vi "Ballard - Arinc-429 RT Driver VI old old.vi"(7 "Operation":T1, 11 "Device Reference in":T2 format="%.0x") -> (0 "Error Code":i32)   [LabVIEW 2016, in "Ballard Arinc-429 Engine.lvlib"]
uses:
  Ballard Arinc-429 Engine.lvlib
  RT Controls/Async Loop Control Enum.ctl
  RT Controls/ReadWrite Selector.ctl
  Shared/Controls and Global/Label.ctl
  Shared/Ballard Arinc-429 Shared.lvlib
  Shared/Controls and Global/transferPeriod.ctl
  <vilib>/NI Veristand/Custom Device API/Data Reference.ctl
  <vilib>/NI Veristand/Custom Device API/Custom Device API.lvlib
  <vilib>/NI Veristand/Custom Device API/Block Data Reference.ctl
  Shared/Controls and Global/Start Bit.ctl
  Shared/Controls and Global/Number of Bits.ctl
  RT Controls/Driver Data.ctl
  RT Controls/RT Label Settings.ctl
  RT Controls/RT HW Channel.ctl
  RT Controls/Error Qs.ctl
  RT Controls/Status Channels Config.ctl
  RT Controls/FIFO.ctl
  RT Controls/Label Transfer Config.ctl
  RT Controls/RT Data.ctl
  RT Controls/RT Param Setting.ctl
  RT Controls/RT Word Settings.ctl
  Shared/Controls and Global/TransferType.ctl
  <vilib>/NI Veristand/Custom Device API/Custom Device Item Ref.ctl
  <vilib>/NI Veristand/Custom Device API/Hardware Interface Driver VI Operation.ctl
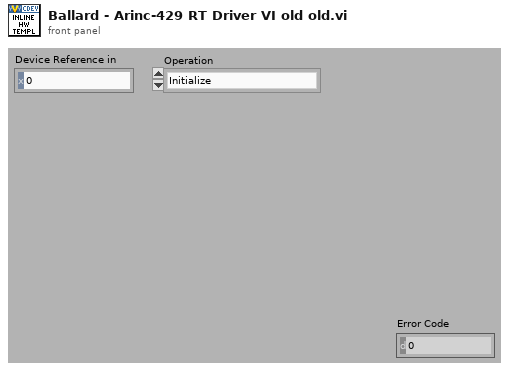
[diagram p1: front panel]
types:
  T1 = typedef "Custom Device API.lvlib/Hardware Interface Driver VI Operation.ctl" = enum16{"Initialize", "Start", "Read Data from HW", "Write Data to HW", "Close"}
  T2 = typedef "Custom Device API.lvlib/Custom Device Item Ref.ctl" = u64
  T3 = typedef "Ballard Arinc-429 Engine.lvlib/RT Data.ctl" = cluster{"HWInput Channels":T4[], "HWOutput Channels":T4[], "board handle":u32, "Start":refnum<notifier>, "HWIn BaseRate":i64, "HWOut BaseRate":i64, "Error Qs":T16, "Error Pub Q":refnum<queue>, "Status Config":T17, "FIFOs":T18, "VI Refs":refnum<vi>[], "Label Transfer Config":T19, "ScheduledSDI":bool}
  T4 = typedef "Ballard Arinc-429 Engine.lvlib/RT HW Channel.ctl" = cluster{"Labels Settings":T5[], "channel handle":u32, "channel #":u16, "Label Map":i32[], "Label Buffer":u32[], "rdBufHandle":u32}
  T5 = typedef "Ballard Arinc-429 Engine.lvlib/RT Label Settings.ctl" = cluster{"Name":string, "xmlName":string, "Label":T6, "transferPeriod":T7, "Driver Data":T8, "SDI_Enabled":bool, "SDI":u8, "Words":T9[], "bufferSize":u32, "RxWordIdx":i32, "TxWordIdx":i32, "TransferType":T15, "has timestamp?":bool}
  T6 = typedef "Ballard Arinc-429 Shared.lvlib/Label.ctl" = u8
  T7 = typedef "Ballard Arinc-429 Shared.lvlib/transferPeriod.ctl" = u32
  T8 = typedef "Ballard Arinc-429 Engine.lvlib/Driver Data.ctl" = cluster{"Lbl Tx Hdl":u32, "Decimation":i32, "IterationOffset":i32, "transfer handle":u32, "RX Word":u32, "TXChange":bool, "RX timestamp":dbl}
  T9 = typedef "Ballard Arinc-429 Engine.lvlib/RT Word Settings.ctl" = cluster{"Block Data Refs":T10[], "Values Array":dbl[], "Length":i32, "FIFO Index":i32, "Param Setting":T12}
  T10 = typedef "Custom Device API.lvlib/Block Data Reference.ctl" = cluster{"Data Reference":T11, "Offset":u64, "Length":u64}
  T11 = typedef "Custom Device API.lvlib/Data Reference.ctl" = i32
  T12 = typedef "Ballard Arinc-429 Engine.lvlib/RT Param Setting.ctl" = cluster{"Start Bit":T13[], "Num Bits":T14[], "Signed?":bool[], "ScaleFac":dbl[], "ScaleOffset":dbl[]}
  T13 = typedef "Ballard Arinc-429 Shared.lvlib/Start Bit.ctl" = i32
  T14 = typedef "Ballard Arinc-429 Shared.lvlib/Number of Bits.ctl" = i32
  T15 = typedef "Ballard Arinc-429 Shared.lvlib/TransferType.ctl" = enum16{"ScheduledLabel", "Acyclic", "Block", "Strobe"}
  T16 = typedef "Ballard Arinc-429 Engine.lvlib/Error Qs.ctl" = cluster{"HWIn":refnum<queue>, "HWOut":refnum<queue>, "TransCfg":refnum<queue>}
  T17 = typedef "Ballard Arinc-429 Engine.lvlib/Status Channels Config.ctl" = cluster{"Error Data Ref":T11, "HWIn Dur Ref":T11, "HWIn Dur Idx":i32, "HWOut Dur Ref":T11, "HWOut Dur Idx":i32}
  T18 = typedef "Ballard Arinc-429 Engine.lvlib/FIFO.ctl" = cluster{"From HWIn":refnum<k33>, "To HWOut":refnum<k33>, "From HWIn Buf":dbl[], "To HWOut Buf":dbl[], "To TansCfg":refnum<k33>, "To TransCfg Buf":dbl[], "From HWOut":refnum<k33>, "From HWOut Buf":dbl[], "Old To HWOut Buf":dbl[]}
  T19 = typedef "Ballard Arinc-429 Engine.lvlib/Label Transfer Config.ctl" = cluster{"Block Data Refs":T10[], "Values Array":dbl[]}
  T20 = typedef "Ballard Arinc-429 Engine.lvlib/Async Loop Control Enum.ctl" = enum16{"Launch", "Start", "Stop"}
  T21 = typedef "Ballard Arinc-429 Engine.lvlib/ReadWrite Selector.ctl" = enum16{"Inline Read", "Inline Write", "Async HWIn", "Async HWOut"}
  T22 = typedef "Ballard Arinc-429 Engine.lvlib/FIFO Idx Qs.ctl" = cluster{"From HWInput":refnum<queue>, "To HWOutput":refnum<queue>, "From HWOutput":refnum<queue>}
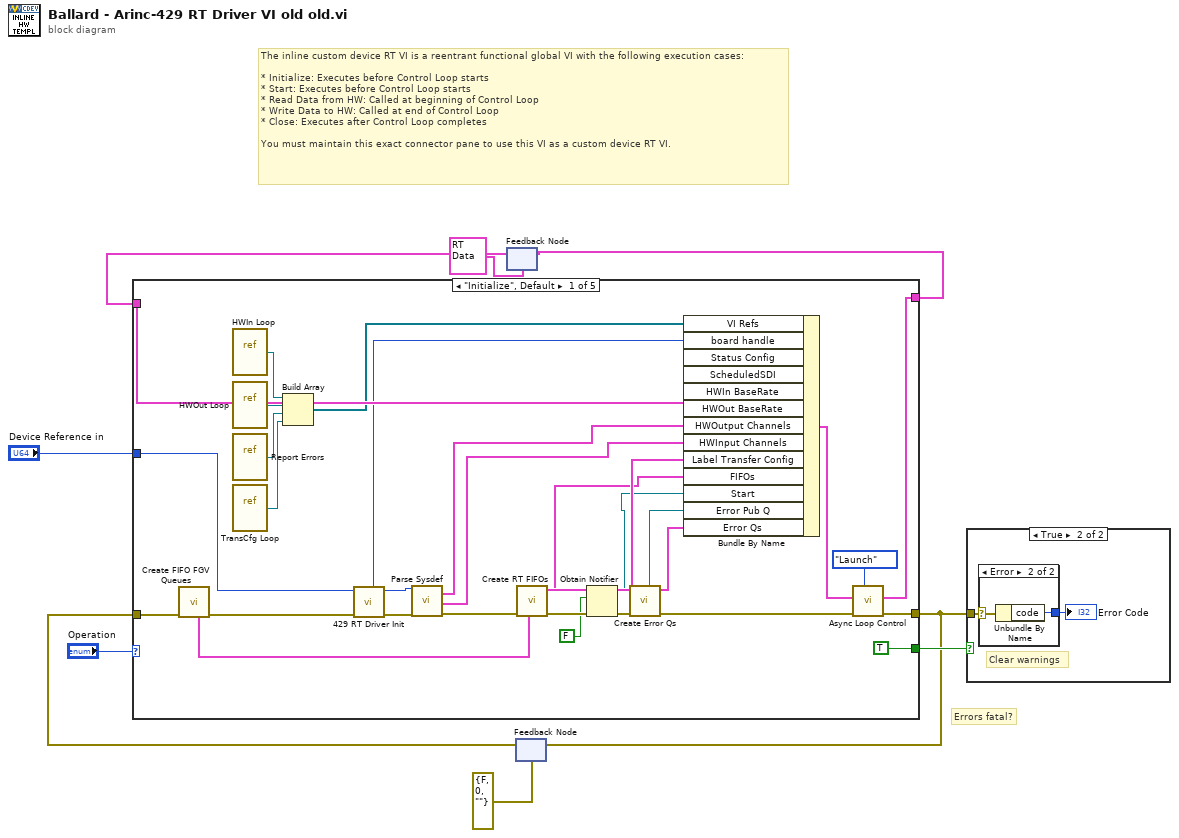
[diagram p0: block diagram]
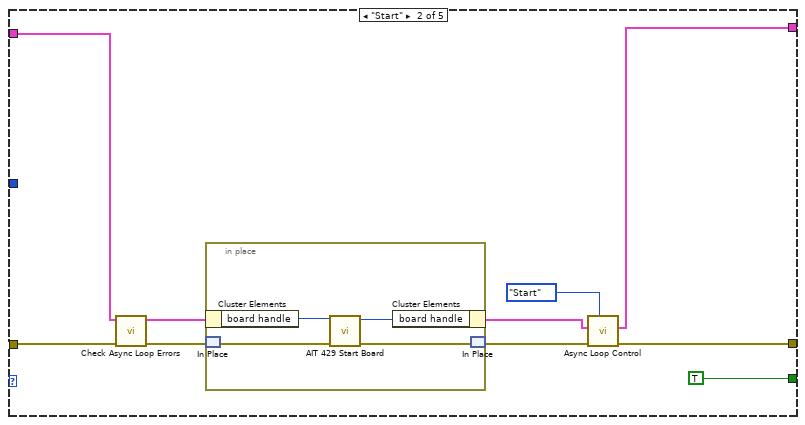
[diagram p4: hidden frame]
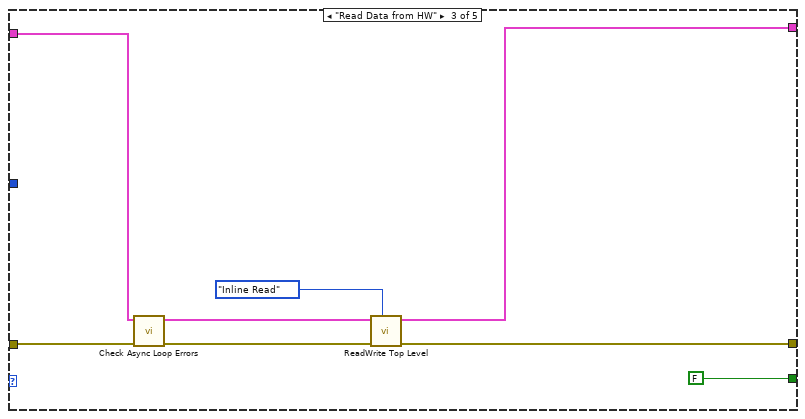
[diagram p5: hidden frame]
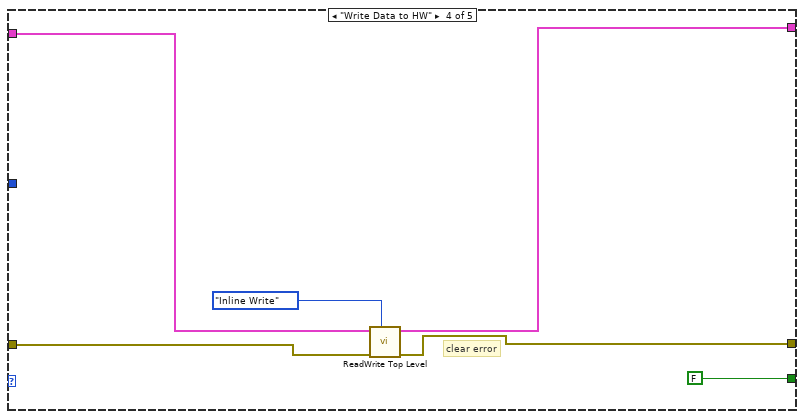
[diagram p6: hidden frame]
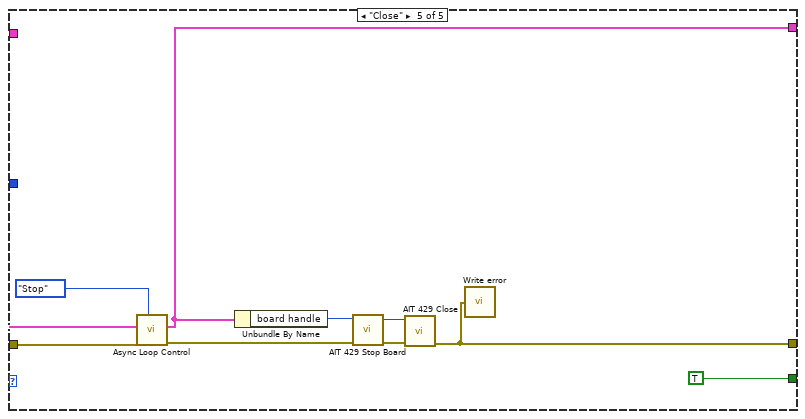
[diagram p7: hidden frame]
diagram:
  # "Errors fatal?"
  # "The inline custom device RT VI is a reentrant functional global VI with the following execution cases:\n\n* Initialize: Executes before Control Loop starts\n* Start: Executes before Control Loop starts\n* Read Data from HW: Called at beginning of Control Loop\n* Write Data to HW: Called at end of Control Loop\n* Close: Executes after Control Loop completes\n\nYou must maintain this exact connector pane to use this VI as a custom device RT VI."
  n1 = feedback #1(T3 {"HWInput Channels"=[], "HWOutput Channels"=[], "board handle"=0, "Start"=refnum, "HWIn BaseRate"=0, "HWOut BaseRate"=0, "Error Qs"={"HWIn"=refnum, "HWOut"=refnum, "TransCfg"=refnum}, "Error Pub Q"=refnum, "Status Config"={"Error Data Ref"=0, "HWIn Dur Ref"=0, "HWIn Dur Idx"=0, "HWOut Dur Ref"=0, "HWOut Dur Idx"=0}, "FIFOs"={"From HWIn"=refnum, "To HWOut"=refnum, "From HWIn Buf"=[], "To HWOut Buf"=[], "To TansCfg"=refnum, "To TransCfg Buf"=[], "From HWOut"=refnum, "From HWOut Buf"=[], "Old To HWOut Buf"=[]}, "VI Refs"=[], "Label Transfer Config"={"Block Data Refs"=[], "Values Array"=[]}, "ScheduledSDI"=FALSE} ("RT Data")) -> (w4:T3)
  n2 = feedback #2(errorcluster {"status"=FALSE, "code"=0, "source"=""} ("error out")) -> (w2:errorcluster)
  n3 = case shown="\"Initialize\", Default" "Operation" {
    tunnel: w4 -> [w29 w51 w62 w71 w76]
    tunnel: "Device Reference in" -> [w31 _ _ _ _]
    tunnel: [w37 w44 w64 w70 w75] -> w3
    tunnel: [w41 w52 w65 w66 w79] -> w1
    tunnel: w2 -> [w11 w50 w59 w69 w78]
    tunnel: [TRUE TRUE FALSE FALSE TRUE] -> w7
    frame "Initialize", Default {
      n4 = call "Create FIFO FGV Queues.vi"("error in (no error)"=w11) -> ("error out"=w13:errorcluster, "FIFO Idx Qs"=w36:T22)  [unwired: 9 in]
      n5 = vi-ref "HWIn Loop.vi"() -> (w33:refnum<vi>)
      n6 = vi-ref "HWOut Loop.vi"() -> (w34:refnum<vi>)
      n7 = vi-ref "Report Errors.vi"() -> (w35:refnum<vi>)
      n8 = vi-ref "TransCfg Loop.vi"() -> (w32:refnum<vi>)
      n9 = Build Array(w33, w34, w35, w32) -> (w27:refnum<vi>[])
      n10 = call "429 RT Driver Init.vi"("error in"=w13, "Device Reference in"=w31) -> ("error out"=w12:errorcluster, "Device Reference out"=w30:T2, "board handle"=w26:u32)  [unwired: 5 in, 2 out]
      n11 = call "Parse Sysdef.vi"("Device Reference in"=w30, "error in (no error)"=w12) -> ("HWOutput Section Data"=w20:T4[], "HWInput Section Data"=w19:T4[], "error out"=w25:errorcluster)  [unwired: 10 in, 5 out]
      n12 = call "Create RT FIFOs.vi"("FIFO Idx Qs"=w36, "error in (no error)"=w25) -> ("error out"=w43:errorcluster, "output cluster"=w17:T18, "Label Transfer Config"=w18:T19)  [unwired: 7 in]
      n13 = Obtain Notifier(notification data type=FALSE, error in (no error)=w43) -> (notifier out=w16:refnum<notifier>, error out=w39:errorcluster)  [unwired: 2 in, 1 out]
      n14 = call "Create Error Qs.vi"("error in (no error)"=w39) -> ("error out"=w10:errorcluster, "Error Qs"=w14:T16, "Error Publishing Q"=w15:refnum<queue>)  [unwired: 8 in]
      n15 = Bundle By Name(cluster=w29, "VI Refs"=w27, "board handle"=w26, "HWOutput Channels"=w20, "HWInput Channels"=w19, "Label Transfer Config"=w18, "FIFOs"=w17, "Start"=w16, "Error Pub Q"=w15, "Error Qs"=w14) -> (w28:T3, "Status Config"=w24:T17, "ScheduledSDI"=w23:bool, "HWIn BaseRate"=w22:i64, "HWOut BaseRate"=w21:i64)
      n16 = call "Async Loop Control.vi"("Action"=Async_Loop_Control_Enum."Launch", "error in (no error)"=w10, "RT Data In"=w28) -> ("error out"=w41:errorcluster, "RT Data Out"=w37:T3)  [unwired: 7 in]
    }
    frame "Start" {
      n17 = call "Check Async Loop Errors.vi"("error in (no error)"=w50, "RT Data in"=w51) -> ("error out"=w48:errorcluster, "RT Data Out"=w47:T3)  [unwired: 8 in]
      n18 = in-place {
        n19 = in-place-cluster #3(w47) -> ("board handle"=w55:u32)
        n20 = in-place-match #4(w48) -> (w57:errorcluster)
        n21 = call <instrlib>:"AIT 429 Start Board.vi"("error in (no error)"=w57, "board handle"=w55) -> ("error out"=w56:errorcluster, "board handle"=w54:u64)  [unwired: 8 in]
        n22 = in-place-cluster #3("board handle"=w54) -> (w46:T3)
        n23 = in-place-match #4(w56) -> (w45:errorcluster)
      }
      n24 = call "Async Loop Control.vi"("Action"=Async_Loop_Control_Enum."Start", "error in (no error)"=w45, "RT Data In"=w46) -> ("error out"=w52:errorcluster, "RT Data Out"=w44:T3)  [unwired: 7 in]
    }
    frame "Read Data from HW" {
      n25 = call "Check Async Loop Errors.vi"("error in (no error)"=w59, "RT Data in"=w62) -> ("error out"=w60:errorcluster, "RT Data Out"=w61:T3)  [unwired: 8 in]
      n26 = call "ReadWrite Top Level.vi"("Mode"=ReadWrite_Selector."Inline Read", "error in (no error)"=w60, "RT Data in"=w61) -> ("error out"=w65:errorcluster, "RT Data out"=w64:T3)  [unwired: 7 in]
    }
    frame "Write Data to HW" {
      # "clear error"
      n27 = call "ReadWrite Top Level.vi"("Mode"=ReadWrite_Selector."Inline Write", "error in (no error)"=w69, "RT Data in"=w71) -> ("error out"=w66:errorcluster, "RT Data out"=w70:T3)  [unwired: 7 in]
    }
    frame "Close" {
      n28 = call "Async Loop Control.vi"("Action"=Async_Loop_Control_Enum."Stop", "error in (no error)"=w78, "RT Data In"=w76) -> ("error out"=w81:errorcluster, "RT Data Out"=w75:T3)  [unwired: 7 in]
      n29 = Unbundle By Name(w75) -> ("board handle"=w74:u32)
      n30 = call <instrlib>:"AIT 429 Stop Board.vi"("error in (no error)"=w81, "board handle"=w74) -> ("error out"=w73:errorcluster, "board handle"=w72:u64)  [unwired: 8 in]
      n31 = call <instrlib>:"AIT 429 Close.vi"("error in (no error)"=w73, "board handle"=w72) -> ("error out"=w79:errorcluster)  [unwired: 9 in]
      n32 = call "Write error.vi"("error in (no error)"=w79) -> ()
    }
  }
  n33 = feedback-in #1(w3) -> ()
  n34 = feedback-in #2(w1) -> ()
  n35 = case shown="True" w7 {
    tunnel: w1 -> [_ w82]
    frame False {
    }
    frame True {
      # "Clear warnings"
      n36 = case shown="Error" w82 {
        selector: w82 -> [_ w85]
        tunnel: [_ w84] -> w83
        frame No Error {
        }
        frame Error {
          n37 = Unbundle By Name(w85) -> ("code"=w84:i32)
        }
      }
      "Error Code" <- w83
    }
  }
